vi "AFM_view_soft.vi"() -> ()   [LabVIEW 2019]
uses:
  <vilib>/Math Plots/3D Math Plots/3D Scatter/3D Scatter XCtrl/3D Scatter.xctl
  <vilib>/Instr/_visa.llb/VISA Configure Serial Port (Instr).vi
  <vilib>/Math Plots/3D Math Plots/3D Scatter/3D Scatter Datatype/Public/Plot Helper (Vector).vi
  <vilib>/Math Plots/3D Math Plots/3D Scatter/3D Scatter Datatype/3D Scatter Datatype.lvclass
  <vilib>/Math Plots/3D Math Plots/3D Plot/3D Plot Datatype/3D Plot Datatype.lvclass
panel:
  out "3D Scatter":refnum<class "3D Plot Datatype.lvclass">[](xcontrol)
  in  "STOP":bool
  out "Read buffer":string
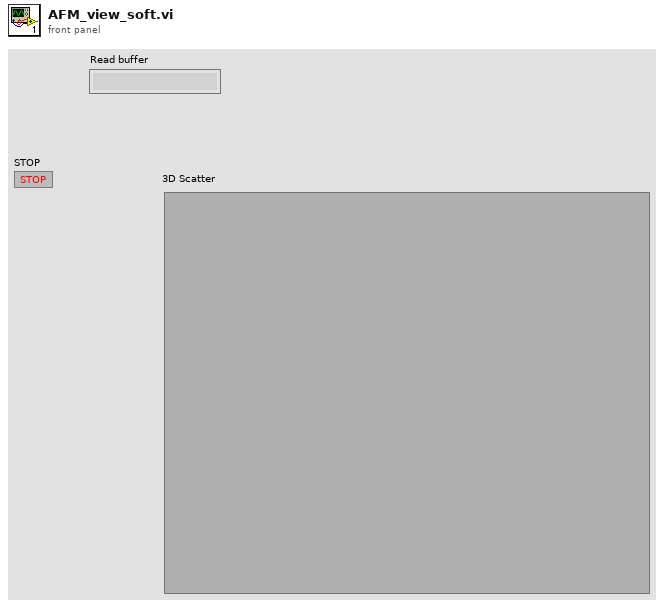
[diagram p1: front panel]
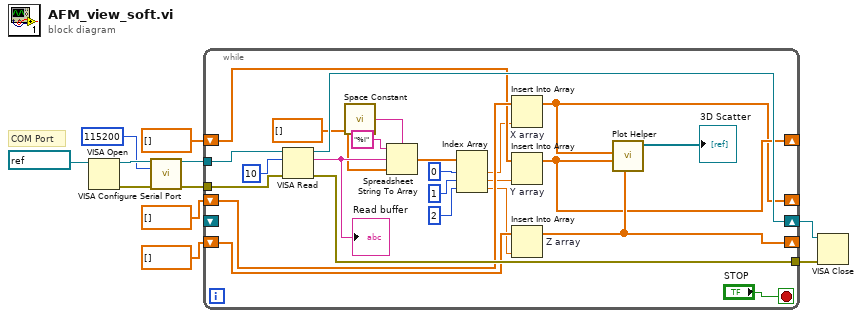
[diagram p0: block diagram]
diagram:
  # "COM Port"
  n1 = VISA Open(VISA resource name=refnum<visa-resource-name> "COM6") -> (VISA resource name=w8:refnum<visa-resource-name>, error out=w6:errorcluster)  [unwired: 4 in]
  n2 = call-poly "VISA Configure Serial Port"("VISA resource name"=w8, "baud rate (9600)"=u32 115200, "error in (no error)"=w6) -> ("VISA resource name out"=w5:refnum<visa-resource-name>, "error out"=w4:errorcluster)  [unwired: 11 in]
  n3 = while {
    tunnel: [w31] -> w10
    shift-right: [w35] -> w11
    shift-left: _ -> [_]
    tunnel: w5 -> [w27]
    tunnel: w4 -> [w26]
    shift-right: [w14] -> _
    shift-left: dbl[] [] -> [w21]
    shift-right: [w12] -> _
    shift-left: dbl[] [] -> [w20]
    shift-right: [w13] -> _
    shift-left: dbl[] [] -> [w19]
    stop <- "STOP" stop-if-true
    n4 = VISA Read(VISA resource name=w27, byte count=u32 10, error in (no error)=w26) -> (VISA resource name out=w35:refnum<visa-resource-name>, read buffer=w25:string, error out=w31:errorcluster)  [unwired: 1 out]
    "Read buffer" <- w25
    n5 = call <vilib>:"Space Constant.vi"() -> ("String"=w22:string)
    n6 = Spreadsheet String To Array(delimiter (Tab)=w22, format string="%i", spreadsheet string=w25, array type (2D Dbl)=dbl[] []) -> (array=w23:dbl[])
    n7 = Index Array(array=w23, index #1=0 ("index (row)"), index #2=1 ("index (row)"), index #3=2 ("index (row)")) -> (element #1=w17:dbl, element #2=w16:dbl, element #3=w15:dbl)
    n8 = Insert Into Array "X array"(array=w20, new element=w17) -> (w12:dbl[])  [unwired: 1 in]
    n9 = Insert Into Array "Y array"(array=w19, new element=w16) -> (w13:dbl[])  [unwired: 1 in]
    n10 = Insert Into Array "Z array"(array=w21, new element=w15) -> (w14:dbl[])  [unwired: 1 in]
    n11 = call-poly <vilib>:"Plot Helper.vi"("z vector"=w14, "y vector"=w13, "x vector"=w12) -> ("3D Plot lvclass Array out"=→"3D Scatter":refnum<class "3D Plot Datatype.lvclass">[])  [unwired: 3 in, 5 out]
  }
  n12 = VISA Close(VISA resource name=w11, error in (no error)=w10) -> ()  [unwired: 1 out]
